vi "init.vi"(8 "error in":errorcluster, 10 "TBM module configuration in":refnum<class "TBM module configuration.lvclass">, 11 "tag bus configurable plugin module in":refnum<class "fixed channel tag bus module.lvclass">) -> (0 "error out":errorcluster, 1 "data allocations":T1, 2 "execution settings":T4, 3 "tag bus configurable plugin module out":refnum<class "fixed channel tag bus module.lvclass">)   [LabVIEW 2013, in "fixed channel tag bus module.lvclass"]
doc: "Provides an interface for initializing a module at runtime. While this interface performs no operations, a child should provide an override which may open any necessary references or sessions, allocate necessary memory, and perform any final configuration validataion before providing the full configuration <b>execution data</b> to the calling process."
uses:
  fixed channel tag bus module.lvclass
  <vilib>/NI/Tag Bus Module Framework/module configuration/TBM module configuration.lvclass
  <vilib>/NI/Tag Bus Module Framework/runtime/execution settings.ctl
  <vilib>/NI/Tag Bus Module Framework/channel/data tables.ctl
  <vilib>/NI/Tag Bus/dictionary/data dictionary.lvclass
  <vilib>/NI/Tag Bus/dictionary table pair.ctl
  <vilib>/NI/Tag Bus/table/data table.ctl
  configuration/fixed channel tag bus module configuration.lvclass
  fixed channel tag bus module.lvclass/fixed channel tag bus module.ctl
  <vilib>/NI/Tag Bus Module Framework/channel/TBM channel.lvclass
  <vilib>/NI/Tag Bus Module Framework/runtime/TBM module execution interface.lvclass
  <vilib>/NI/Tag Bus Data Framework/Configuration Editor/PL Framework Configuration Tool.lvlib
  <vilib>/NI/Tag Bus/tag bus.lvlib
  <vilib>/NI/Tag Bus/table/data table.lvlib
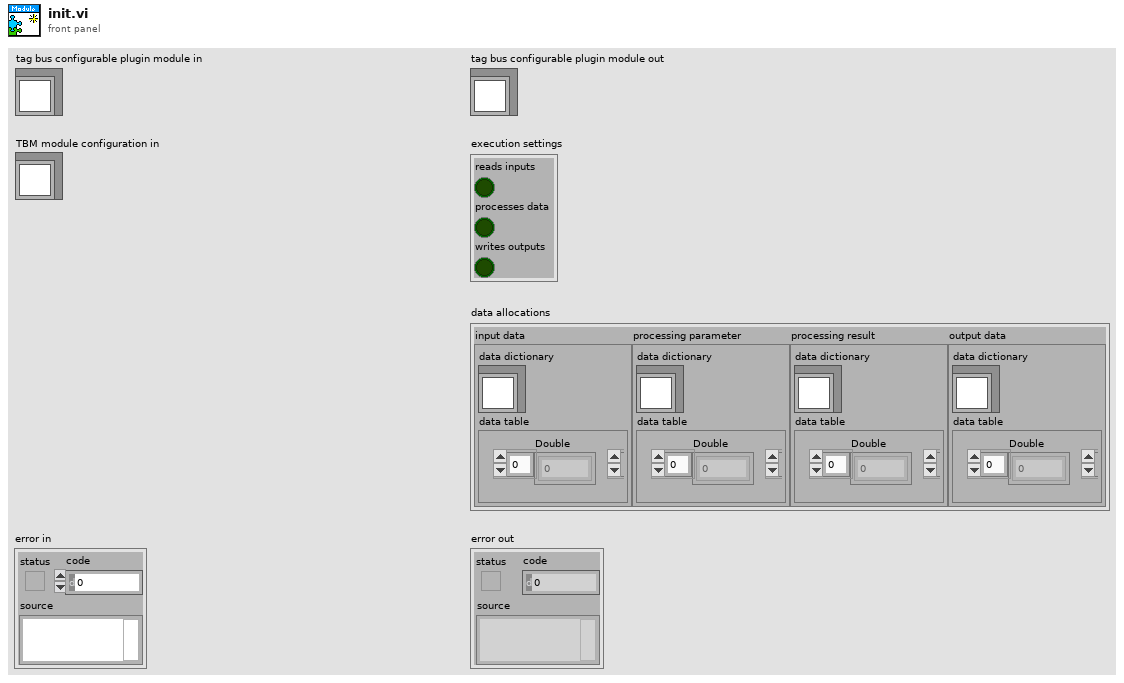
[diagram p1: front panel]
types:
  T1 = typedef "TBM channel.lvclass/data tables.ctl" = cluster{"input data":T2, "processing parameter":T2, "processing result":T2, "output data":T2}
  T2 = typedef "tag bus.lvlib/dictionary table pair.ctl" = cluster{"data dictionary":refnum<class "data dictionary.lvclass">, "data table":T3}
  T3 = typedef "tag bus.lvlib/data table.lvlib/data table.ctl" = cluster{"Double":dbl[], "Single":sgl[], "I64":i64[], "I32":i32[], "I16":i16[], "I8":i8[], "U64":u64[], "U32":u32[], "U16":u16[], "U8":u8[], "Boolean":bool[], "String":string[], "Array of Double":cluster{"DBL Array":dbl[]}[], "Array of Single":cluster{"SGL Array":sgl[]}[], "Array of I64":cluster{"I64 Array":i64[]}[], "Array of I32":cluster{"I32 Array":i32[]}[], "Array of I16":cluster{"I16 Array":i16[]}[], "Array of I8":cluster{"I8 Array":i8[]}[], "Array of U64":cluster{"U64 Array":u64[]}[], "Array of U32":cluster{"U32 Array":u32[]}[], "Array of U16":cluster{"U16 Array":u16[]}[], "Array of U8":cluster{"U8 Array":u8[]}[], "Array of Boolean":cluster{"Boolean Array":bool[]}[], "Array of String":cluster{"String Array":string[]}[]}
  T4 = typedef "TBM module execution interface.lvclass/execution settings.ctl" = cluster{"reads inputs":bool, "processes data":bool, "writes outputs":bool}
  T5 = typedef "Channel Run Time Mapping Info.ctl" = cluster{"Channel Indicies":i32[], "Channel Names":string[]}
  T6 = typedef "fixed channel tag bus module.lvclass/inputs.ctl" = cluster{"placeholder":i32}
  T7 = typedef "fixed channel tag bus module.lvclass/parameters.ctl" = cluster{"placeholder":i32}
  T8 = typedef "fixed channel tag bus module.lvclass/results.ctl" = cluster{"placeholder":i32}
  T9 = typedef "fixed channel tag bus module.lvclass/outputs.ctl" = cluster{"placeholder":i32}
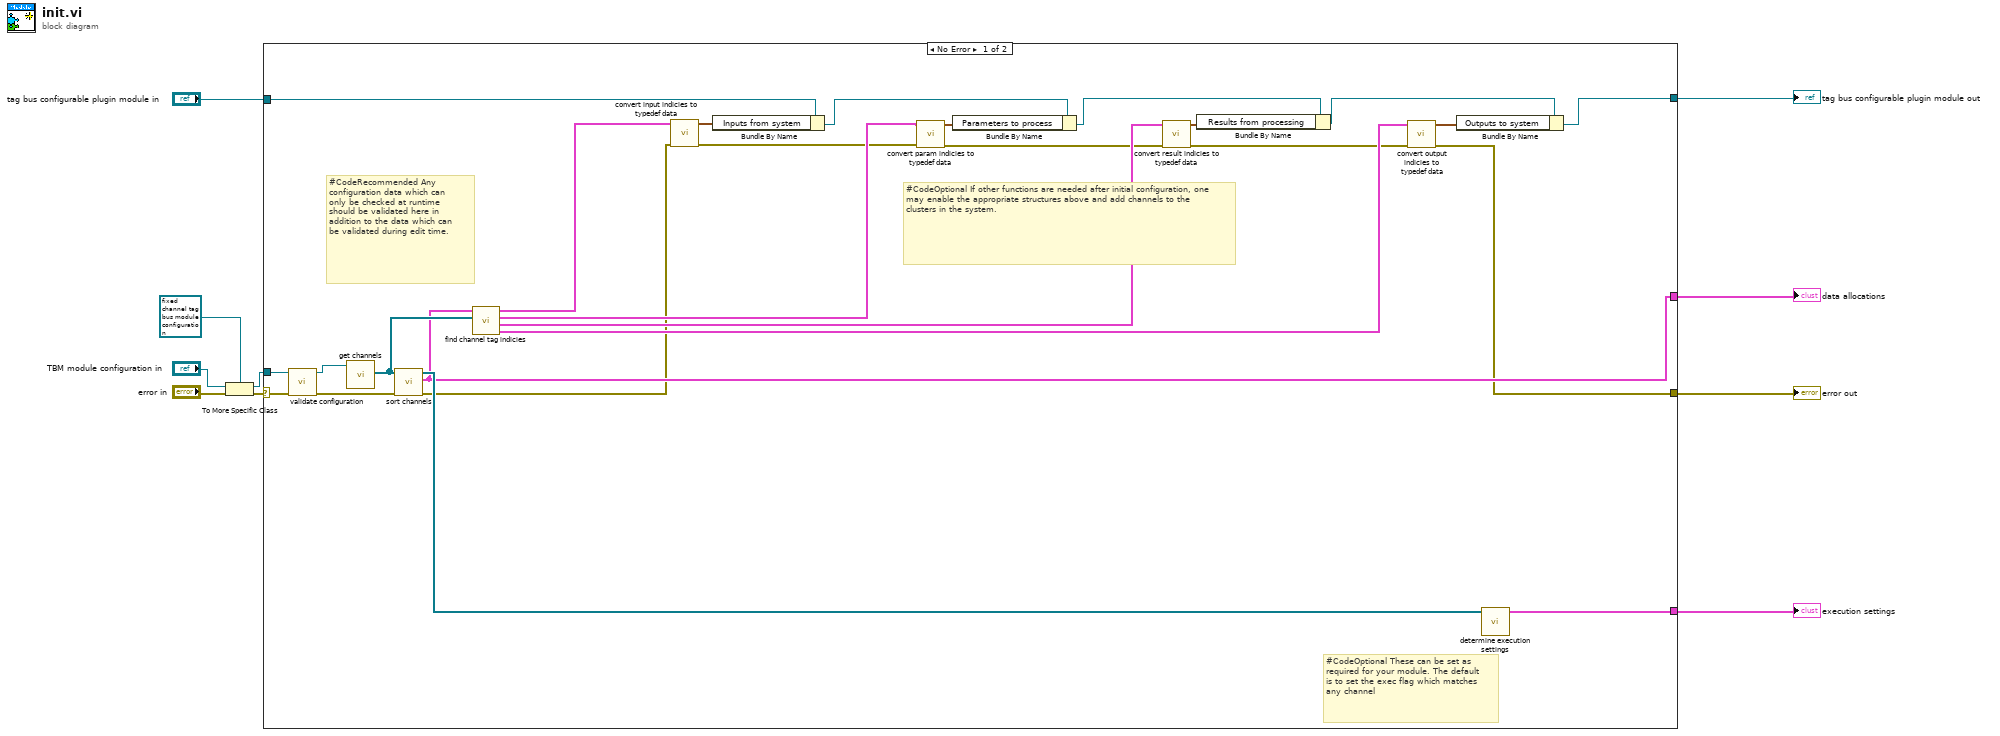
[diagram p0: block diagram]
diagram:
  n1 = To More Specific Class(target class=refnum<class "fixed channel tag bus module configuration.lvclass"> refnum ("Synchronous module configuration"), reference="TBM module configuration in", error in="error in") -> (specific class reference=w1:refnum<class "fixed channel tag bus module configuration.lvclass">, error out=w2:errorcluster)
  n2 = case shown="No Error" w2 {
    selector: w2 -> [w34 w37]
    tunnel: w1 -> [w33 _]
    tunnel: "tag bus configurable plugin module in" -> [w28 w38]
    tunnel: [w20 w38] -> w8
    tunnel: [w11 w37] -> w7
    tunnel: [w29 _] -> w5
    tunnel: [w36 _] -> w6
    frame No Error {
      # "#CodeOptional If other functions are needed after initial configuration, one may enable the appropriate structures above and add channels to the clusters in the system."
      # "#CodeRecommended Any configuration data which can only be checked at runtime should be validated here in addition to the data which can be validated during edit time."
      # "#CodeOptional These can be set as required for your module. The default is to set the exec flag which matches any channel"
      n3 = call-dynamic "validate configuration.vi"("error in"=w34, "tag bus configurable plugin module configuration in"=w33) -> ("error out"=w35:errorcluster, "tag bus configurable plugin module configuration out"=w32:refnum<class "fixed channel tag bus module configuration.lvclass">)  [unwired: 8 in]
      n4 = call-dynamic "get channels.vi"("user tag bus module configuration In"=w32) -> ("channels"=w30:refnum<class "TBM channel.lvclass">[])  [unwired: 9 in, 1 out]
      n5 = call <vilib>:"sort channels.vi"("error in"=w35, "channels in"=w30) -> ("error out"=w12:errorcluster, "data allocations"=w29:T1, "channels out"=w31:refnum<class "TBM channel.lvclass">[])  [unwired: 7 in]
      n6 = call <vilib>:"find channel tag indicies.vi"("channels"=w30, "data allocations"=w29) -> ("Output Indicies"=w21:T5, "Result Indicies"=w24:T5, "Parameter Indicies"=w25:T5, "Input Indicies"=w27:T5)  [unwired: 6 in]
      n7 = call "convert input indicies to typedef data.vi"("error in"=w12, "Input Channel Mapping info"=w27) -> ("error out"=w15:errorcluster, "Inputs from system"=w19:T6)  [unwired: 8 in]
      n8 = Bundle By Name(cluster=w28, "Inputs from system"=w19) -> (w26:refnum<class "fixed channel tag bus module.lvclass">)
      n9 = call "convert param indicies to typedef data.vi"("error in"=w15, "Parameter Mapping Info"=w25) -> ("error out"=w14:errorcluster, "Parameters to process"=w18:T7)  [unwired: 8 in]
      n10 = Bundle By Name(cluster=w26, "Parameters to process"=w18) -> (w23:refnum<class "fixed channel tag bus module.lvclass">)
      n11 = call "convert result indicies to typedef data.vi"("error in"=w14, "Result Mapping Info"=w24) -> ("error out"=w13:errorcluster, "Results from processing"=w17:T8)  [unwired: 8 in]
      n12 = Bundle By Name(cluster=w23, "Results from processing"=w17) -> (w22:refnum<class "fixed channel tag bus module.lvclass">)
      n13 = call "convert output indicies to typedef data.vi"("error in"=w13, "Output Mapping Info"=w21) -> ("error out"=w11:errorcluster, "Outputs to system"=w16:T9)  [unwired: 8 in]
      n14 = Bundle By Name(cluster=w22, "Outputs to system"=w16) -> (w20:refnum<class "fixed channel tag bus module.lvclass">)
      n15 = call <vilib>:"determine execution settings.vi"("channels"=w31) -> ("execution settings"=w36:T4)  [unwired: 10 in]
    }
    frame Error {
    }
  }
  "error out" <- w7
  "tag bus configurable plugin module out" <- w8
  "execution settings" <- w6
  "data allocations" <- w5
